vi "temp calc.vi"(11 "Numeric":dbl format="%#_13g") -> (3 "x/y":dbl)   [LabVIEW 2016]
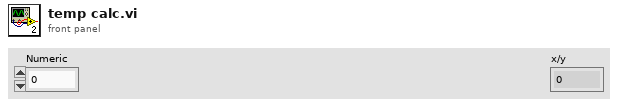
[diagram p1: front panel]
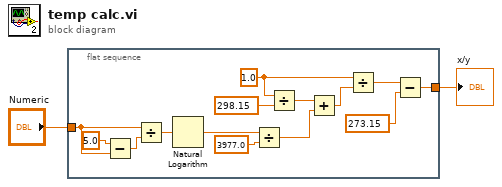
[diagram p0: block diagram]
diagram:
  n1 = flat-sequence {
    tunnel: "Numeric" -> [w6]
    tunnel: [w3] -> w1
    frame #0 {
      w14 = 1.0
      n2 = Subtract(x=5.0, y=w6) -> (x-y=w12:dbl)
      n3 = Divide(x=w6, y=w12) -> (x/y=w11:dbl)
      n4 = Natural Logarithm(1:w11) -> (0:w10:dbl)
      n5 = Divide(x=w10, y=3977.0) -> (x/y=w8:dbl)
      n6 = Divide(x=w14, y=298.15) -> (x/y=w9:dbl)
      n7 = Add(x=w9, y=w8) -> (x+y=w7:dbl)
      n8 = Divide(x=w14, y=w7) -> (x/y=w5:dbl)
      n9 = Subtract(x=w5, y=273.15) -> (x-y=w3:dbl)
    }
  }
  "x/y" <- w1
